vi "IV hysteresis V4.vi"() -> ()   [LabVIEW 2014]
uses:
  Environmental Chamber LabVIEW and Instruments/Drivers and Software/LabVIEW 8.2 Drivers/keithley_24xx/Keithley 24XX/Public/Data/Read (Single Point).vi
  <vilib>/Utility/file.llb/Write To Spreadsheet File (string).vi
  Environmental Chamber LabVIEW and Instruments/Drivers and Software/keithley_24xx/Keithley 24XX/Keithley 24XX.lvlib
panel:
  out "Current cycle":dbl
  out "Runtime (min)":dbl
  in  "voltage settings 3":T1={"V (V)"=0.1, "steps"=4.0, "cycles"=1, "Reverse scan"=FALSE} {"cycles" min=1 max=10000}
  out "Points to sweep (V)":dbl[](array[numeric])
  in  "RUN":bool
  in  "Delay between points (s)":dbl[](array[numeric])
  out "Runtime (hrs)":dbl
  out "Sweep rate (V/s)":dbl[](array[numeric])
  out "Bias (V)":dbl
  out "Delay (s)":dbl
  out "File path":path
  out "2420 IV curve":cluster{"X":dbl[], "Y":dbl[]}[](graph)
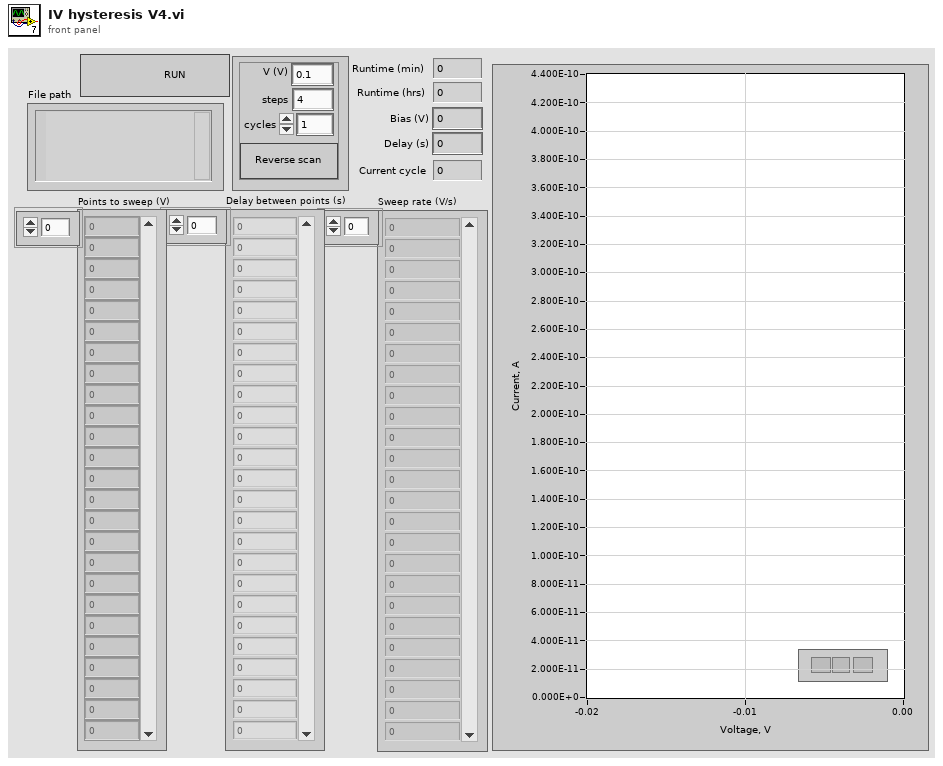
[diagram p1: front panel]
types:
  T1 = cluster{"V (V)":dbl, "steps":dbl, "cycles":u32, "Reverse scan":bool}
  T2 = enum16{"open", "open or create", "create or replace", "create", "open (read only)"}
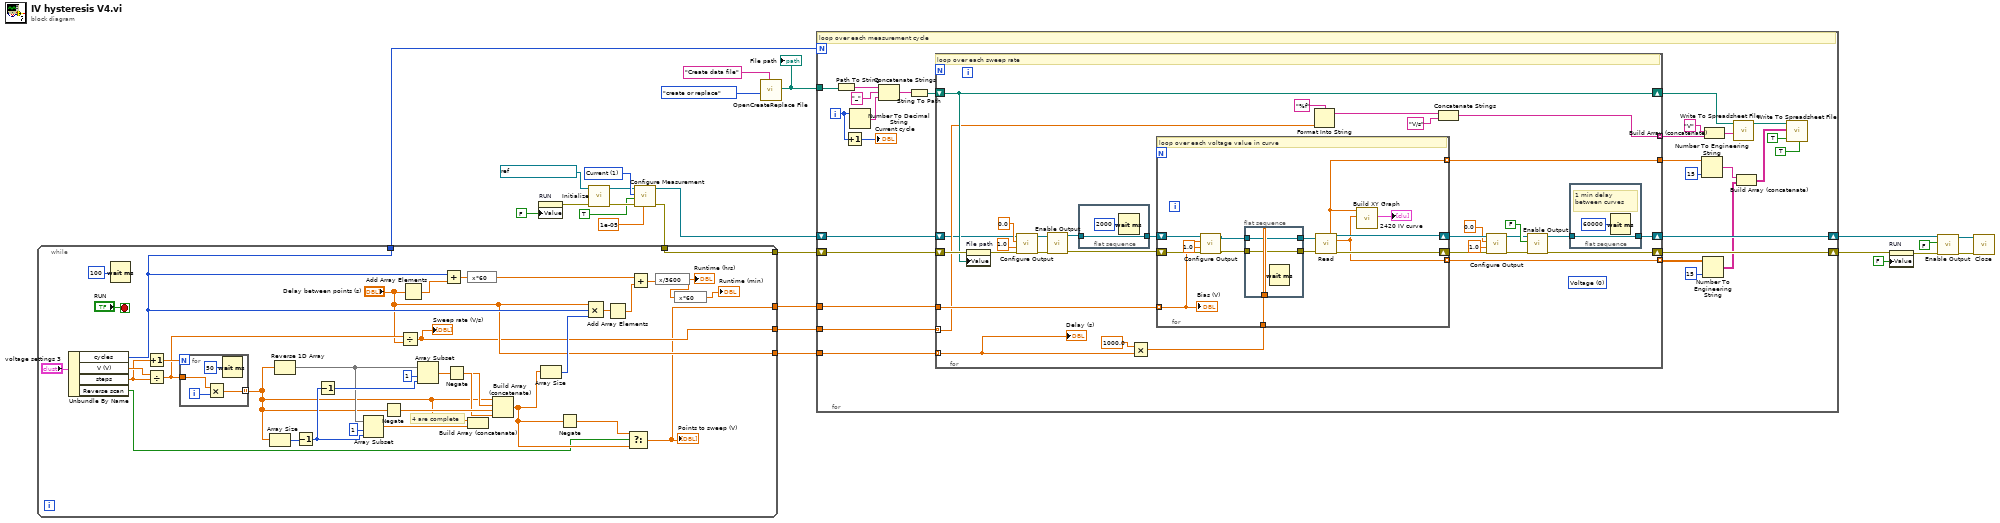
[diagram p0: block diagram]
diagram:
  w18 = u16 1 items=["Volts", "Current", "Resistance"] ("Function (0: Volts)")
  n1 = property on="RUN" class="Bool (strict)"("Value"=FALSE ("RUN")) -> (error out=w9:errorcluster)  [unwired: 2 in, 1 out]
  n2 = call "Initialize.vi"("error in (no error)"=w9, "VISA resource name"=refnum<visa-resource-name> "GPIB1::24::INSTR") -> ("error out"=w16:errorcluster, "VISA resource name out"=w17:refnum<visa-resource-name>)  [unwired: 8 in]
  n3 = call "Configure Measurement.vi"("Manual Range (1.0)"=1e-05, "error in (no error)"=w16, "Enable Auto Range (T:Enable)"=TRUE, "Function (0: Volts)"=w18, "VISA resource name"=w17) -> ("error out"=w12:errorcluster, "VISA resource name out"=w21:refnum<visa-resource-name>)  [unwired: 5 in]
  n4 = while {
    tunnel: w12 -> [w46]
    tunnel: [w46] -> w11
    tunnel: [w45] -> w8
    tunnel: ["Delay between points (s)"] -> w7
    tunnel: [w34] -> w6
    tunnel: [w35] -> w5
    stop <- "RUN" stop-if-true
    # "4 are complete"
    n5 = Unbundle By Name("voltage settings 3") -> ("cycles"=w45:u32, "V (V)"=w57:dbl, "steps"=w56:dbl, "Reverse scan"=w28:bool)
    n6 = Wait (ms)(milliseconds to wait=u32 100) -> ()  [unwired: 1 out]
    n7 = Increment(x=w56) -> (x+1=w55:dbl)
    n8 = Divide(x=w57, y=w56) -> (x/y=w47:dbl)
    n9 = for {
      N: w55 -> [_]
      tunnel: w47 -> [w64]
      tunnel: [w61] -> w30 mode=indexing
      i -> [w63]
      n10 = Multiply(x=w64, y=w63) -> (x*y=w61:dbl)
      n11 = Wait (ms)(milliseconds to wait=u32 50) -> ()  [unwired: 1 out]
    }
    n12 = Array Size(array=w30) -> (size(s)=w42:i32)
    n13 = Reverse 1D Array(array=w30) -> (reversed array=w37:dbl[])
    n14 = Decrement(x=w42) -> (x-1=w36:i32)
    n15 = Decrement(x=w36) -> (x-1=w41:i32)
    n16 = Array Subset(array=w37, index=1, length=w36) -> (w29:dbl[])
    n17 = Negate(x=w30) -> (-x=w40:dbl[])
    n18 = Divide(x=w47, y="Delay between points (s)") -> (x/y=w35:dbl[])
    "Sweep rate (V/s)" <- w35
    n19 = Add Array Elements(numeric array="Delay between points (s)") -> (sum=w50:dbl)
    n20 = Array Subset(array=w37, index=1, length=w41) -> (w31:dbl[])
    n21 = Add(x=w45, y=w50) -> (x+y=w53:dbl)
    n22 = Negate(x=w31) -> (-x=w39:dbl[])
    n23 = expression code="x*60"(w53) -> (w49:dbl)
    n24 = Build Array (concatenate)(w30, w29) -> ()  [unwired: 1 out]
    n25 = Build Array (concatenate)(w30, w31, w40, w39) -> (w33:dbl[])
    n26 = Array Size(array=w33) -> (size(s)=w51:i32)
    n27 = Negate(x=w33) -> (-x=w32:dbl[])
    n28 = Compound Arithmetic op=MULTIPLY("Delay between points (s)", w45, w51) -> (w54:dbl[])
    n29 = Add Array Elements(numeric array=w54) -> (sum=w48:dbl)
    n30 = Select(t=w32, s=w28, f=w33) -> (s? t:f=w34:dbl[])
    "Points to sweep (V)" <- w34
    n31 = Add(x=w49, y=w48) -> (x+y=w52:dbl)
    n32 = expression code="x/3600"(w52) -> (w27:dbl)
    "Runtime (hrs)" <- w27
    n33 = expression code="x*60"(w27) -> (→"Runtime (min)":dbl)
  }
  n34 = call "OpenCreateReplace File.vi"("prompt"="Create data file", "function (open:0)"=T2."create or replace") -> ("new file path"=w1:path)  [unwired: 6 in, 3 out]
  "File path" <- w1
  n35 = for {
    N: w8 -> [_]
    tunnel: w5 -> [w93]
    tunnel: w6 -> [w92]
    tunnel: w7 -> [w79]
    tunnel: w1 -> [w68]
    shift-right: [w91] -> w22
    shift-left: w21 -> [w90]
    shift-right: [w81] -> w3
    shift-left: w11 -> [w80]
    i -> [w66]
    # "loop over each measurement cycle"
    n36 = Path To String(path=w68) -> (string=w78:string)
    n37 = Increment(x=w66) -> (x+1=→"Current cycle":i32)
    n38 = Number To Decimal String(number=w66) -> (decimal integer string=w76:string)  [unwired: 1 in]
    n39 = Concatenate Strings(w78, "_" ("string"), w76) -> (w77:string)
    n40 = String To Path(string=w77) -> (path=w67:path)
    n41 = for {
      shift-right: [w103] -> w81
      shift-left: w80 -> [w118]
      shift-right: [w121] -> w91
      shift-left: w90 -> [w99]
      shift-right: [w117] -> w88
      shift-left: w67 -> [w117]
      tunnel: [w123] -> w85 mode=indexing
      tunnel: w93 -> [w114] mode=indexing
      tunnel: w92 -> [w122]
      tunnel: w79 -> [w112] mode=indexing
      tunnel: [w120] -> w73 mode=indexing
      tunnel: [w119] -> w70
      (unwired) u16 0 items=["Voltage", "Current"] ("Source Mode  (0: Voltage)")
      # "loop over each sweep rate"
      n42 = property on="File path" class="Path"(error in=w118, "Value"=w117) -> (error out=w98:errorcluster)  [unwired: 1 in, 1 out]
      n43 = call "Configure Output.vi"("error in (no error)"=w98, "Compliance  Level (0.1)"=1.0, "Output Level (0)"=0.0, "VISA resource name"=w99) -> ("error out"=w95:errorcluster, "VISA resource name out"=w97:refnum<visa-resource-name>)  [unwired: 6 in]
      n44 = call "Enable Output.vi"("error in (no error)"=w95, "VISA resource name"=w97) -> ("error out"=w94:errorcluster, "VISA resource name out"=w96:refnum<visa-resource-name>)  [unwired: 8 in]
      n45 = flat-sequence {
        tunnel: [w126] -> w100
        tunnel: w96 -> [w126]
        frame #0 {
          # "delay between curves"
          n46 = Wait (ms)(milliseconds to wait=u32 2000 ("value")) -> ()  [unwired: 1 out]
        }
      }
      n47 = Multiply(x=1000.0 ("Manual Range (1.0)"), y=w112) -> (x*y=w116:dbl)
      n48 = for {
        shift-right: [w140] -> w109
        shift-left: w94 -> [w139]
        shift-right: [w141] -> w110
        shift-left: w100 -> [w138]
        tunnel: w116 -> [w134]
        tunnel: w122 -> [w133] mode=indexing
        tunnel: [w132] -> w120 mode=indexing
        tunnel: [w131] -> w119 mode=indexing
        # "loop over each voltage value in curve"
        n49 = call "Configure Output.vi"("error in (no error)"=w139, "Compliance  Level (0.1)"=1.0, "Output Level (0)"=w133, "VISA resource name"=w138) -> ("error out"=w128:errorcluster, "VISA resource name out"=w129:refnum<visa-resource-name>)  [unwired: 6 in]
        n50 = flat-sequence {
          tunnel: [w144] -> w137
          tunnel: w129 -> [w144]
          tunnel: w128 -> [w143]
          tunnel: [w143] -> w136
          tunnel: w134 -> [w142]
          frame #0 {
            n51 = Wait (ms)(milliseconds to wait=w142) -> ()  [unwired: 1 out]
          }
        }
        n52 = call-poly "Read.vi"("VISA resource name"=w137, "error in (no error)"=w136) -> ("Voltage"=w131:sgl, "VISA resource name out"=w141:refnum<visa-resource-name>, "Current"=w132:sgl, "error out"=w140:errorcluster)  [unwired: 7 in, 3 out]
        n53 = call "Build XY Graph"("Y Input"=w132, "X Input"=w131) -> ("XY Graph"=→"2420 IV curve":cluster{"X":dbl[], "Y":dbl[]}[])  [unwired: 8 in, 1 out]
        "Bias (V)" <- w133
      }
      n54 = Format Into String(format string="%f", w114) -> (resulting string=w113:string)  [unwired: 2 in, 1 out]
      n55 = Concatenate Strings(w113, "V/s" ("string")) -> (w123:string)
      n56 = call "Configure Output.vi"("error in (no error)"=w109, "Compliance  Level (0.1)"=1.0, "Output Level (0)"=0.0, "VISA resource name"=w110) -> ("error out"=w104:errorcluster, "VISA resource name out"=w106:refnum<visa-resource-name>)  [unwired: 6 in]
      n57 = call "Enable Output.vi"("error in (no error)"=w104, "Enable Output (T: Enable)"=FALSE, "VISA resource name"=w106) -> ("error out"=w103:errorcluster, "VISA resource name out"=w105:refnum<visa-resource-name>)  [unwired: 7 in]
      n58 = flat-sequence {
        tunnel: w105 -> [w145]
        tunnel: [w145] -> w121
        frame #0 {
          # "1 min delay between curves"
          n59 = Wait (ms)(milliseconds to wait=u32 60000 ("value")) -> ()  [unwired: 1 out]
        }
      }
      "Delay (s)" <- w112
    }
    n60 = Number To Engineering String(2:i16 15 ("precision (6)"), 4:w70) -> (0:w69:string[])  [unwired: 2 in]
    n61 = Number To Engineering String(2:i16 15 ("precision (6)"), 4:w73) -> (0:w72:string[][])  [unwired: 2 in]
    n62 = Build Array (concatenate)("V", w85) -> (w84:string[])
    n63 = call-poly <vilib>:"Write To Spreadsheet File.vi"("1D data"=w84, "file path (dialog if empty)"=w88) -> ("new file path (Not A Path if cancelled)"=w87:path)  [unwired: 6 in]
    n64 = Build Array (concatenate)(w69, w72) -> (w83:string[][])
    n65 = call-poly <vilib>:"Write To Spreadsheet File.vi"("transpose? (no:F)"=TRUE, "append to file? (new file:F)"=TRUE ("transpose? (no:F)"), "2D data"=w83, "file path (dialog if empty)"=w87) -> ()  [unwired: 4 in, 1 out]
  }
  n66 = property on="RUN" class="Bool (strict)"(error in=w3, "Value"=FALSE ("RUN")) -> (error out=w2:errorcluster)  [unwired: 1 in, 1 out]
  n67 = call "Enable Output.vi"("error in (no error)"=w2, "Enable Output (T: Enable)"=FALSE, "VISA resource name"=w22) -> ("error out"=w23:errorcluster, "VISA resource name out"=w25:refnum<visa-resource-name>)  [unwired: 7 in]
  n68 = call "Close.vi"("error in (no error)"=w23, "VISA resource name"=w25) -> ()  [unwired: 9 in, 1 out]
